vi "HypervisorFinalWriteAndClose.vi"(8 "ErrorIn":errorcluster, 11 "QIn":refnum<queue>) -> (0 "ErrorOut":errorcluster)   [LabVIEW 2018]
doc: "This VI calls for the final logging of any remaining events in the Hypervisor loop and then closes the Queue.\n\n\nCopyright © 2019 Epimedia, Inc. All Rights Reserved.\n\nThe Epimedia Application Library is Copyright © 2009-2017 Epimedia, Inc. \nAll Rights Reserved. Used under license."
uses:
  Queue/HyperVisor.ctl
  <vilib>/Utility/sysdir.llb/System Directory Type.ctl
panel:
  # "Copyright © 2019 Epimedia, Inc. All Rights Reserved.\n\nThe Epimedia Application Library is Copyright © 2009-2017 Epimedia, Inc. \nAll Rights Reserved. Used under license."
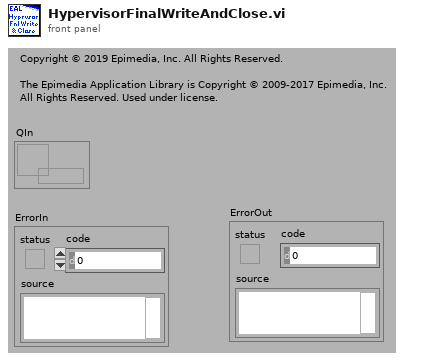
[diagram p1: front panel]
types:
  T1 = typedef "System Directory Type.ctl" = i32
  T2 = typedef "HyperVisor.ctl" = cluster{"TimeOut":dbl, string, "Data":variant, "StopHpvsr":bool}
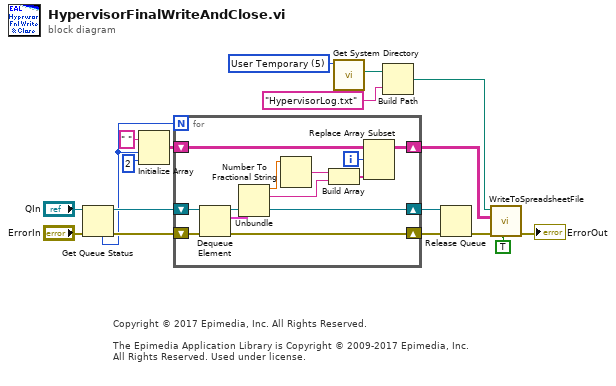
[diagram p0: block diagram]
diagram:
  w13 = T1 5 items=["User Home"=0, "User Desktop"=1, "User Documents"=2, "User Application Data"=3, "User Preferences"=4, "User Temporary"=5, "Public Documents"=6, "Public Application Data"=7, "Public Preferences"=8, "Public Cache"=13, "System Core Libraries"=9, "System Installed Libraries"=10, "Application Files"=11, "Boot Volume Root"=12] ("system directory type")
  # "Copyright © 2017 Epimedia, Inc. All Rights Reserved.\n\nThe Epimedia Application Library is Copyright © 2009-2017 Epimedia, Inc. \nAll Rights Reserved. Used under license."
  n1 = Get Queue Status(queue="QIn", error in (no error)="ErrorIn") -> (queue out=w8:refnum<queue>, error out=w6:errorcluster, # elements in queue=w1:i32)  [unwired: 1 in, 5 out]
  n2 = Initialize Array(" ", w1, 2 ("dimension size")) -> (w15:string[][])
  n3 = for {
    N: w1 -> [_]
    shift-right: [w24] -> w14
    shift-left: w15 -> [w30]
    shift-right: [w23] -> w5
    shift-left: w8 -> [w21]
    shift-right: [w19] -> w4
    shift-left: w6 -> [w22]
    i -> [w25]
    n4 = Dequeue Element(queue=w21, error in (no error)=w22) -> (queue out=w23:refnum<queue>, element=w20:T2, error out=w19:errorcluster)  [unwired: 2 out]
    n5 = Unbundle(w20) -> ("TimeOut"=w29:dbl, w28:string)  [unwired: 2 out]
    n6 = Number To Fractional String(number=w29) -> (F-format string=w27:string)  [unwired: 1 in, 2 out]
    n7 = Build Array(w27, w28) -> (w26:string[])
    n8 = Replace Array Subset(array=w30, new element=w26, index (row)=w25) -> (w24:string[][])  [unwired: 1 in]
  }
  n9 = call <vilib>:"Get System Directory.vi"("system directory type"=w13) -> ("system directory"=w12:path)  [unwired: 10 in]
  n10 = Build Path(base path=w12, name or relative path="HypervisorLog.txt") -> (appended path=w10:path)
  n11 = Release Queue(queue=w5, error in (no error)=w4) -> (error out=w3:errorcluster)  [unwired: 1 in, 2 out]
  n12 = call "WriteToSpreadsheetFile.vi"("Append?(NewFile:F)"=TRUE ("append to file? (new file:F)"), "ErrorIn"=w3, "2D-Data"=w14, "FilePath(DialogIfEmpty)"=w10) -> ("ErrorOut"=→"ErrorOut":errorcluster)  [unwired: 4 in, 3 out]
